vi "Data Bundle.vi"(8 "Error In":errorcluster, 11 "InterfaceData":T1 {"GenEast"."TotalFuel(L)" format="%.2f"; "GenEast"."FuelRate(L/H)" format="%.2f"; "GenEast"."ApparentPower(VA)" format="%.2f"; "GenEast"."BattVoltage(V)" format="%.2f"; "GenEast"."Freq(Hz)" format="%.2f"; "GenEast"."RunHours(hr)" format="%.2f"; "GenEast"."PowerFactor" format="%.2f"; "GenEast"."ReactivePower(VAR)" format="%.2f"; "GenEast"."ActivePower(W)" format="%.2f"; "GenWest"."TotalFuel(L)" format="%.2f"; "GenWest"."FuelRate(L/H)" format="%.2f"; "GenWest"."ApparentPower(VA)" format="%.2f"; "GenWest"."BattVoltage(V)" format="%.2f"; "GenWest"."Freq(Hz)" format="%.2f"; "GenWest"."RunHours(hr)" format="%.2f"; "GenWest"."PowerFactor" format="%.2f"; "GenWest"."ReactivePower(VAR)" format="%.2f"; "GenWest"."ActivePower(W)" format="%.2f"; "Converter Alarms 2" format="%016b"; "Converter Faults 2" format="%016b"; "Controller Faults" format="%016b"; "System Status" format="%016b"; "Converter Alarms 1" format="%016b"; "Converter Faults 1" format="%016b"; "Solar Faults" format="%016b"; "ES Rack 10 Alarms" format="%016b"; "ES Rack 9 Alarms" format="%016b"; "ES Rack 8 Alarms" format="%016b"; "ES Rack 7 Alarms" format="%016b"; "ES Rack 6 Alarms" format="%016b"; "ES Rack 5 Alarms" format="%016b"; "ES Rack 4 Alarms" format="%016b"; "ES Rack 3 Alarms" format="%016b"; "ES Rack 2 Alarms" format="%016b"; "ES Rack 1 Alarms" format="%016b"; "ES System Alarms" format="%016b"; "System Faults" format="%016b"; "ES Rack 10 Faults" format="%016b"; "ES Rack 9 Faults" format="%016b"; "ES Rack 8 Faults" format="%016b"; "ES Rack 7  Faults" format="%016b"; "ES Rack 6 Faults" format="%016b"; "ES Rack 5 Faults" format="%016b"; "ES Rack 4 Faults" format="%016b"; "ES Rack 3 Faults" format="%016b"; "ES Rack 2 Faults" format="%016b"; "ES Rack 1 Faults" format="%016b"; "ES System Faults" format="%016b"}) -> (0 "Error Out":errorcluster, 3 "Data Out":string[](array[string]))   [LabVIEW 2014]
uses:
  Controls/Interface Data.ctl
  Controls/Gen Data.ctl
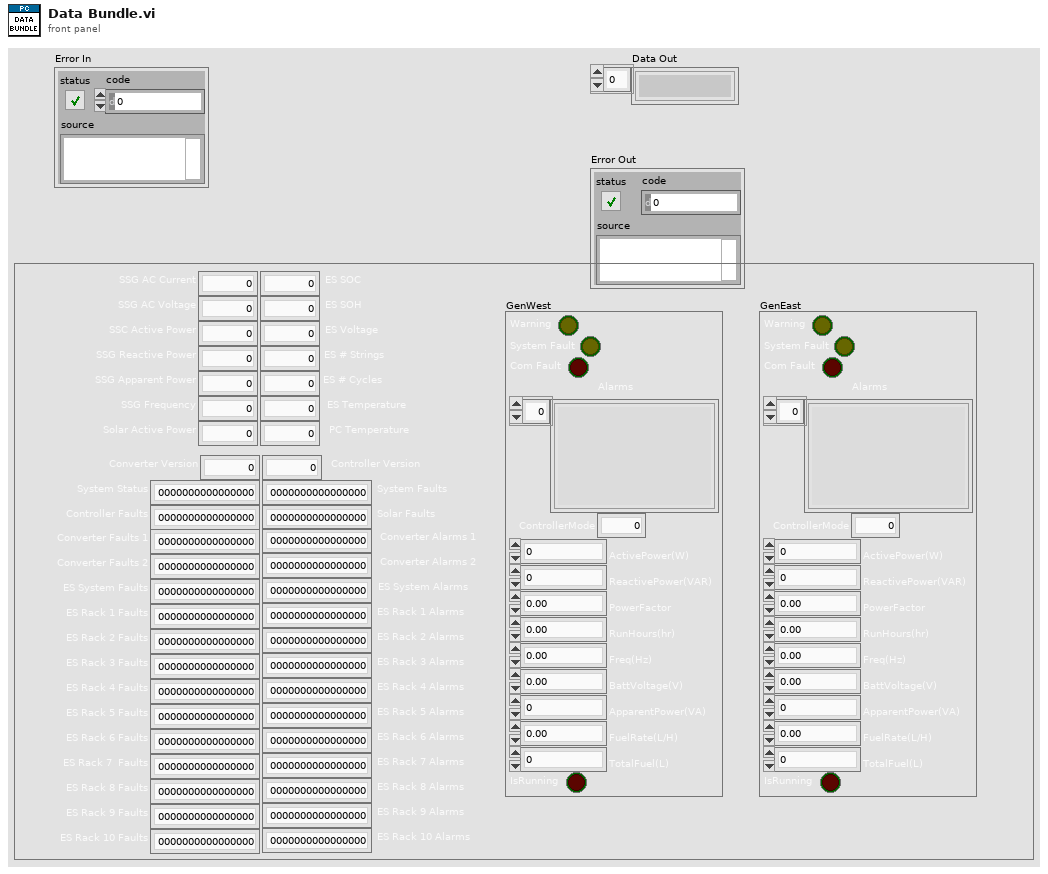
[diagram p1: front panel]
types:
  T1 = typedef "Interface Data.ctl" = cluster{"SSG AC Current":i16, "SSG AC Voltage":i16, "SSC Active Power":i16, "SSG Reactive Power":i16, "SSG Apparent Power":i16, "SSG Frequency":i16, "ES SOC":i16, "ES SOH":i16, "ES Voltage":i16, "ES # Strings":i16, "ES # Cycles":i16, "ES Temperature":i16, "PC Temperature":i16, "Solar Active Power":i16, "Converter Version":i16, "Controller Version":i16, "System Status":i16, "System Faults":i16, "Controller Faults":i16, "ES System Faults":i16, "ES System Alarms":i16, "Converter Faults 1":i16, "Converter Faults 2":i16, "Converter Alarms 1":i16, "Converter Alarms 2":i16, "Solar Faults":i16, "ES Rack 1 Faults":i16, "ES Rack 2 Faults":i16, "ES Rack 3 Faults":i16, "ES Rack 4 Faults":i16, "ES Rack 5 Faults":i16, "ES Rack 6 Faults":i16, "ES Rack 7  Faults":i16, "ES Rack 8 Faults":i16, "ES Rack 9 Faults":i16, "ES Rack 10 Faults":i16, "ES Rack 1 Alarms":i16, "ES Rack 2 Alarms":i16, "ES Rack 3 Alarms":i16, "ES Rack 4 Alarms":i16, "ES Rack 5 Alarms":i16, "ES Rack 6 Alarms":i16, "ES Rack 7 Alarms":i16, "ES Rack 8 Alarms":i16, "ES Rack 9 Alarms":i16, "ES Rack 10 Alarms":i16, "GenWest":T2, "GenEast":T2}
  T2 = typedef "Gen Data.ctl" = cluster{"Warning":bool, "System Fault":bool, "Com Fault":bool, "Alarms":string[], "ControllerMode":u16, "ActivePower(W)":i32, "ReactivePower(VAR)":i32, "PowerFactor":dbl, "RunHours(hr)":dbl, "Freq(Hz)":dbl, "BattVoltage(V)":dbl, "ApparentPower(VA)":i32, "FuelRate(L/H)":dbl, "TotalFuel(L)":u32, "IsRunning":bool}
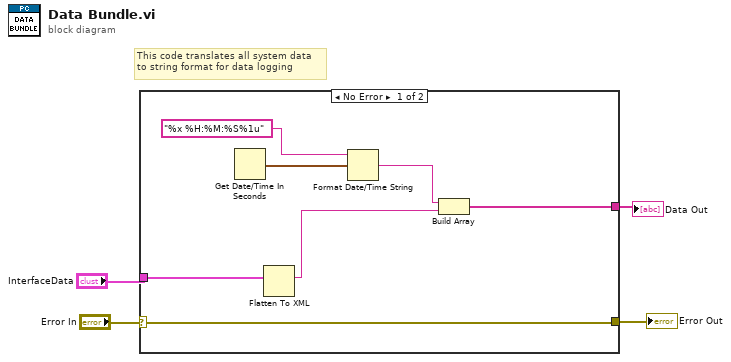
[diagram p0: block diagram]
diagram:
  # "This code translates all system data \nto string format for data logging"
  n1 = case shown="No Error" "Error In" {
    selector: "Error In" -> [w9 w12]
    tunnel: [w9 w12] -> w3
    tunnel: "InterfaceData" -> [w7 _]
    tunnel: [w5 _] -> w1
    frame No Error {
      n2 = Get Date/Time In Seconds() -> (seconds since 1Jan1904=w10:timestamp)
      n3 = Flatten To XML(anything=w7) -> (xml string=w6:string)
      n4 = Format Date/Time String(time format string (%c)="%x %H:%M:%S%1u", seconds (now)=w10) -> (date/time string=w8:string)  [unwired: 1 in]
      n5 = Build Array(w8, w6) -> (w5:string[])
    }
    frame Error {
    }
  }
  "Data Out" <- w1
  "Error Out" <- w3
